vi "LCB Get Dev Type Name.vi"(8 "error in (no error)":errorcluster caption="Fehler (Eingang, kein Fehler)", 11 "Device Handle":i64) -> (0 "error out":errorcluster caption="Fehler (Ausgang)", 3 "Device Type":string)   [LabVIEW 2021, in "labbCAN_Bus_API.lvlib"]
doc: "LCB_Func long __stdcall LCB_GetDevTypeName(dev_hdl hDev,\n char *pNameStringBuf,\n int StringBufSize);"
uses:
  labbCAN_Bus_API.lvlib
  labbCAN_Bus_API.dll
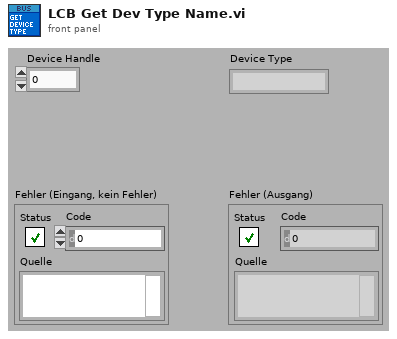
[diagram p1: front panel]
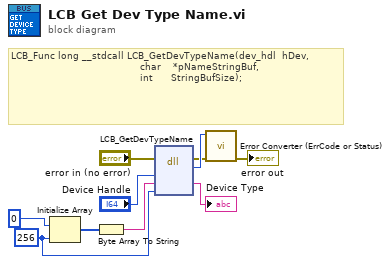
[diagram p0: block diagram]
diagram:
  w1 = 256 ("Dimension")
  # "LCB_Func long __stdcall LCB_GetDevTypeName(dev_hdl  hDev,\n                                           char    *pNameStringBuf,\n                                           int      StringBufSize);"
  n1 = Initialize Array(u8 0 ("Element"), w1) -> (w9:u8[])
  n2 = Byte Array To String(unsigned byte array=w9) -> (string=w8:string)
  n3 = dll-call lib="C:/GIT/DensityGradientProject/CETONI_SDK/labbCAN_Bus_API.*" fn="LCB_GetDevTypeName"(error in="error in (no error)", "hDev"="Device Handle", "pNameStringBuf"=w8, "StringBufSize"=w1) -> (error out=w3:errorcluster, "Rückgabetyp"=w4:i32, "pNameStringBuf"=→"Device Type":string)  [unwired: 4 in, 1 out]
  n4 = call "Error Converter (ErrCode or Status).vi"("error in (no error)"=w3, "error code"=w4) -> ("error out"=→"error out":errorcluster)  [unwired: 9 in]
